vi "GetItemInfo.vi"(8 "error in (no error)":errorcluster, 11 "Array":cluster{"Name":string, "Value":string}[](array[cluster])) -> (0 "error out":errorcluster, 2 "item":T1, 3 "Value":string)   [LabVIEW 2014, in "OPCUA XML(dev).lvlib"]
uses:
  OPCUA XML(dev).lvlib
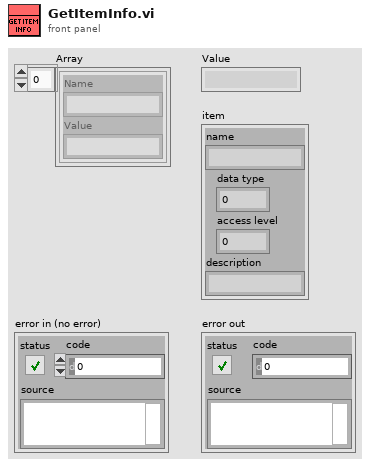
[diagram p1: front panel]
types:
  T1 = cluster{"name":string, "data type":u16, "access level":u16, "description":string}
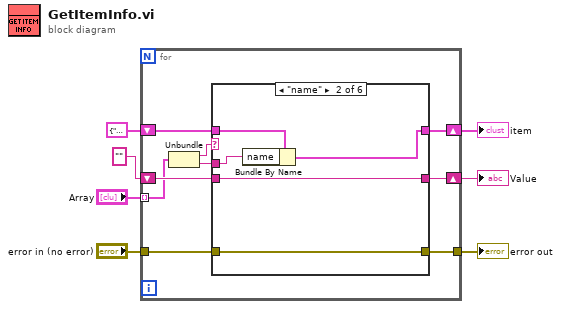
[diagram p0: block diagram]
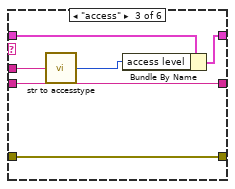
[diagram p3: hidden frame]
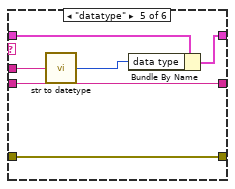
[diagram p5: hidden frame]
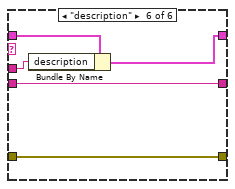
[diagram p6: hidden frame]
diagram:
  n1 = for {
    tunnel: "error in (no error)" -> [w12]
    shift-right: [w15] -> w7
    shift-left: T1 {"name"="", "data type"=1, "access level"=1, "description"=""} ("item") -> [w16]
    shift-right: [w14] -> w6
    shift-left: "" ("Value") -> [w13]
    tunnel: "Array" -> [w11] mode=indexing
    tunnel: [w8] -> w5
    n2 = Unbundle(w11) -> ("Name"=w10:string, "Value"=w9:string)
    n3 = case shown="\"name\"" w10 {
      tunnel: [w19 w24 w30 w32 w39 w44] -> w8
      tunnel: w12 -> [w19 w24 w30 w32 w39 w44]
      tunnel: w16 -> [w17 w23 w29 w33 w38 w43]
      tunnel: [w17 w22 w28 w33 w37 w42] -> w15
      tunnel: [w18 w21 w26 w31 w35 w41] -> w14
      tunnel: w13 -> [w18 w21 w26 w31 w35 w41]
      tunnel: w9 -> [_ w20 w25 _ w34 w40]
      frame Default {
      }
      frame "name" {
        n4 = Bundle By Name(cluster=w23, "name"=w20) -> (w22:T1)
      }
      frame "access" {
        n5 = call "str to accesstype.vi"("String"=w25) -> ("access level"=w27:u16)  [unwired: 6 in]
        n6 = Bundle By Name(cluster=w29, "access level"=w27) -> (w28:T1)
      }
      frame "initialValue" {
      }
      frame "datatype" {
        n7 = call "str to datetype.vi"("String"=w34) -> ("data type"=w36:u16)  [unwired: 5 in, 1 out]
        n8 = Bundle By Name(cluster=w38, "data type"=w36) -> (w37:T1)
      }
      frame "description" {
        n9 = Bundle By Name(cluster=w43, "description"=w40) -> (w42:T1)
      }
    }
  }
  "item" <- w7
  "Value" <- w6
  "error out" <- w5
